vi "Find_Reference.vi"(3 "error in (no error)":errorcluster, 4 "Label":string="Pilot", 5 "Cluster in":refnum<vi>) -> (0 "error out":errorcluster, 1 "Ctl Refnum":refnum<vi>)   [LabVIEW 2023]
doc: "Find the control/ind reference by the name/label"
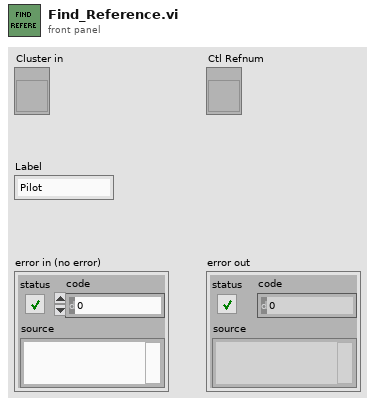
[diagram p1: front panel]
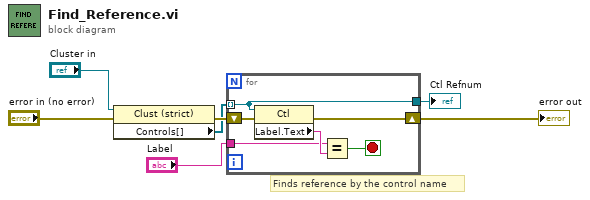
[diagram p0: block diagram]
diagram:
  # "Finds reference by the control name"
  n1 = property class="Clust (strict)"(reference="Cluster in", error in="error in (no error)") -> (error out=w7:errorcluster, "Controls[]"=w4:refnum<vi>[])  [unwired: 1 out]
  n2 = for {
    tunnel: w4 -> [w11] mode=indexing
    tunnel: [w11] -> w1
    shift-right: [w10] -> w6
    shift-left: w7 -> [w9]
    tunnel: "Label" -> [w8]
    stop <- w12 stop-if-true
    n3 = property class="Ctl"(reference=w11, error in=w9) -> (error out=w10:errorcluster, "Label.Text"=w13:string)  [unwired: 1 out]
    n4 = Equal?(x=w8, y=w13) -> (x = y?=w12:bool)
  }
  "error out" <- w6
  "Ctl Refnum" <- w1
